vi "Initialize.vi"(8 "error in":errorcluster, 10 "InstanceName":string, 11 "Chiller Cluster - 2 Channel.lvclass":refnum<class "Cycler Cluster - 2 Channel.lvclass">) -> (0 "error out":errorcluster, 3 "output cluster":refnum<class "Cycler Cluster - 2 Channel.lvclass">)   [LabVIEW 2023, in "Cycler Cluster - 2 Channel.lvclass"]
uses:
  Cycler Cluster - 2 Channel.lvclass
  Cycler Cluster - 2 Channel.lvclass/Cycler Cluster - 2 Channel.ctl
  aa699e23-44e5-4879-a6c3-559a5ef9d2df.vi
  f052ae29-6a80-40ba-948a-362e912d77bd.vi
  293d8571-9b14-4487-9d38-5c4ef123197a.vi
  16278833-8dfa-4f0a-81f5-f65bd27da24d.vi
  da48c8f8-b897-4dcf-9451-5b341042a248.vi
  f0f9fcd1-ad99-4552-afb1-31be6853704b.vi
  aa699e23-44e5-4879-a6c3-559a5ef9d2df.vi/4bc1c15b-36ab-481f-b8dd-c64075ce723a.vi
  f052ae29-6a80-40ba-948a-362e912d77bd.vi/4bc1c15b-36ab-481f-b8dd-c64075ce723a.vi
  293d8571-9b14-4487-9d38-5c4ef123197a.vi/4bc1c15b-36ab-481f-b8dd-c64075ce723a.vi
  16278833-8dfa-4f0a-81f5-f65bd27da24d.vi/4bc1c15b-36ab-481f-b8dd-c64075ce723a.vi
  da48c8f8-b897-4dcf-9451-5b341042a248.vi/4bc1c15b-36ab-481f-b8dd-c64075ce723a.vi
  f0f9fcd1-ad99-4552-afb1-31be6853704b.vi/4bc1c15b-36ab-481f-b8dd-c64075ce723a.vi
  <vilib>/ADAS Replay HIL/AdasHilServices/AdasHilServices Fill In Error Info Ex.vi
  Utilities/Utilities.lvlib
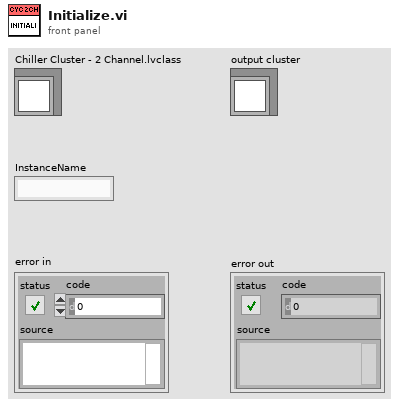
[diagram p1: front panel]
types:
  T1 = cluster{"OnOff.ACT":bool, "ErrorAcknowledge.ACT":bool, "IsoMeasurement.ACT":bool, "ParallelMode.ACT":bool}
  T2 = cluster{"OnOff.STS":i32, "Error.STS":i32, "Watchdog.STS":i32, "IsoMeasurement.STS":i32, "ParallelMode.STS":i32}
  T3 = cluster{"ErrorAcknowledge.ch01.ACT":bool, "OutputEnable.ch01.ACT":bool, "ControlMode.ch01.CTL":u16, "Voltage.ch01.SP":dbl, "VoltageMIN.ch01.SP":dbl, "VoltageMAX.ch01.SP":dbl, "VoltageGrad.ch01.SP":dbl, "Current.ch01.SP":dbl, "CurrentMIN.ch01.SP":dbl, "CurrentMAX.ch01.SP":dbl, "CurrentGrad.ch01.SP":dbl, "Power.ch01.SP":dbl, "Power.ch01.SP":dbl, "Power.ch01.SP":dbl, "PowerGrad.ch01.SP":dbl, "ParameterSet.ch01.CTL":i32}
  T4 = cluster{"Error.ch01.STS":i32, "OutputEnable.ch01.STS":i32, "ControlMode.ch01.STS":u16, "Voltage.ch01.AV":dbl, "Current.ch01.AV":dbl, "Power.ch01.AV":dbl, "VoltageNominal.ch01.AV":dbl, "CurrentNominal.ch01.AV":dbl, "PowerNominal.ch01.AV":dbl, "ParameterSet.ch01.STS":i32}
  T5 = cluster{"ErrorAcknowledge.ch02.ACT":bool, "OutputEnable.ch02.ACT":bool, "ControlMode.ch02.CTL":u16, "Voltage.ch02.SP":dbl, "VoltageMIN.ch02.SP":dbl, "VoltageMAX.ch02.SP":dbl, "VoltageGrad.ch02.SP":dbl, "Current.ch02.SP":dbl, "CurrentMIN.ch02.SP":dbl, "CurrentMAX.ch02.SP":dbl, "CurrentGrad.ch02.SP":dbl, "Power.ch02.SP":dbl, "PowerMIN.ch02.SP":dbl, "PowerMAX.ch02.SP":dbl, "PowerGrad.ch02.SP":dbl, "ParameterSet.ch02.CTL":i32}
  T6 = cluster{"Error.ch02.STS":i32, "OutputEnable.ch02.STS":i32, "ControlMode.ch02.STS":u16, "Voltage.ch02.AV":dbl, "Current.ch02.AV":dbl, "Power.ch02.AV":dbl, "VoltageNominal.ch02.AV":dbl, "CurrentNominal.ch02.AV":dbl, "PowerNominal.ch02.AV":dbl, "ParameterSet.ch02.STS":i32}
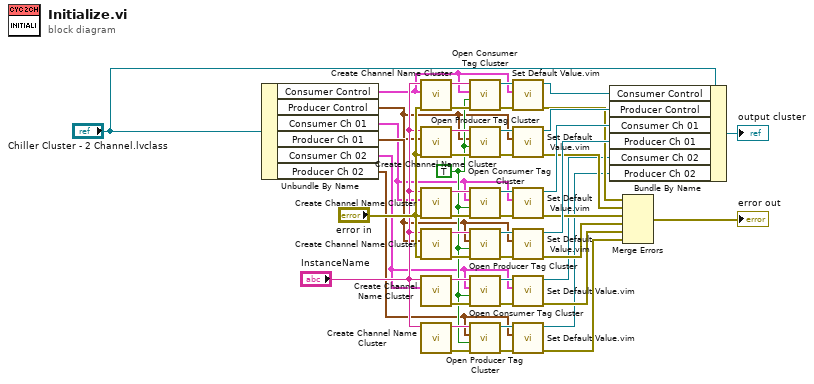
[diagram p0: block diagram]
diagram:
  w12 = TRUE ("Create if not found? (T)")
  n1 = Unbundle By Name("Chiller Cluster - 2 Channel.lvclass") -> ("Consumer Control"=w1:T1, "Producer Control"=w2:T2, "Consumer Ch 01"=w3:T3, "Producer Ch 01"=w4:T4, "Consumer Ch 02"=w5:T5, "Producer Ch 02"=w6:T6)
  n2 = call "Create Channel Name Cluster.vi"("error in"="error in", "Cluster"=w1, "Instance Name"="InstanceName") -> ("error out"=w29:errorcluster, "Data Channel Name"=w48:string)  [unwired: 7 in]
  n3 = call "Create Channel Name Cluster.vi"("error in"="error in", "Cluster"=w2, "Instance Name"="InstanceName") -> ("error out"=w30:errorcluster, "Data Channel Name"=w47:string)  [unwired: 7 in]
  n4 = call "Create Channel Name Cluster.vi"("error in"="error in", "Cluster"=w3, "Instance Name"="InstanceName") -> ("error out"=w35:errorcluster, "Data Channel Name"=w40:string)  [unwired: 7 in]
  n5 = call "Create Channel Name Cluster.vi"("error in"="error in", "Cluster"=w4, "Instance Name"="InstanceName") -> ("error out"=w33:errorcluster, "Data Channel Name"=w39:string)  [unwired: 7 in]
  n6 = call "Create Channel Name Cluster.vi"("Cluster"=w5, "Instance Name"="InstanceName") -> ("error out"=w18:errorcluster, "Data Channel Name"=w14:string)  [unwired: 8 in]
  n7 = call "Create Channel Name Cluster.vi"("Instance Name"="InstanceName") -> ("error out"=w16:errorcluster, "Data Channel Name"=w21:string)  [unwired: 9 in]
  n8 = call "Open Consumer Tag Cluster.vi"("error in"=w29, "Create if not found? (T)"=w12, "Cluster"=w1, "Channel Name"=w48) -> ("error out"=w44:errorcluster, "ADAS HIL Channel"=w46:refnum<k21>)  [unwired: 6 in]
  n9 = call "Open Producer Tag Cluster.vi"("error in"=w30, "Create if not found? (T)"=w12, "Cluster"=w2, "Channel Name"=w47) -> ("error out"=w43:errorcluster, "ADAS HIL Channel"=w42:refnum<k21>)  [unwired: 6 in]
  n10 = call "Open Consumer Tag Cluster.vi"("error in"=w35, "Create if not found? (T)"=w12, "Cluster"=w3, "Channel Name"=w40) -> ("error out"=w36:errorcluster, "ADAS HIL Channel"=w37:refnum<k21>)  [unwired: 6 in]
  n11 = call "Open Producer Tag Cluster.vi"("error in"=w33, "Create if not found? (T)"=w12, "Cluster"=w4, "Channel Name"=w39) -> ("error out"=w34:errorcluster, "ADAS HIL Channel"=w38:refnum<k21>)  [unwired: 6 in]
  n12 = call "Open Consumer Tag Cluster.vi"("error in"=w18, "Create if not found? (T)"=w12, "Cluster"=w5, "Channel Name"=w14) -> ("error out"=w19:errorcluster, "ADAS HIL Channel"=w13:refnum<k21>)  [unwired: 6 in]
  n13 = call "Open Producer Tag Cluster.vi"("error in"=w16, "Create if not found? (T)"=w12, "Cluster"=w6, "Channel Name"=w21) -> ("error out"=w17:errorcluster, "ADAS HIL Channel"=w20:refnum<k21>)  [unwired: 6 in]
  n14 = call "Set Default Value.vim"("error in"=w44, "Data in"=w1, "ADAS HIL Channel in"=w46) -> ("error out"=w27:errorcluster, "ADAS HIL Channel out"=w45:refnum<k21>)  [unwired: 7 in]
  n15 = call "Set Default Value.vim"("error in"=w43, "Data in"=w2, "ADAS HIL Channel in"=w42) -> ("error out"=w26:errorcluster, "ADAS HIL Channel out"=w41:refnum<k21>)  [unwired: 7 in]
  n16 = call "Set Default Value.vim"("error in"=w36, "Data in"=w3, "ADAS HIL Channel in"=w37) -> ("error out"=w25:errorcluster, "ADAS HIL Channel out"=w32:refnum<k21>)  [unwired: 7 in]
  n17 = call "Set Default Value.vim"("error in"=w34, "Data in"=w4, "ADAS HIL Channel in"=w38) -> ("error out"=w24:errorcluster, "ADAS HIL Channel out"=w31:refnum<k21>)  [unwired: 7 in]
  n18 = call "Set Default Value.vim"("error in"=w19, "Data in"=w5, "ADAS HIL Channel in"=w13) -> ("error out"=w11:errorcluster, "ADAS HIL Channel out"=w9:refnum<k21>)  [unwired: 7 in]
  n19 = call "Set Default Value.vim"("error in"=w17, "Data in"=w6, "ADAS HIL Channel in"=w20) -> ("error out"=w10:errorcluster, "ADAS HIL Channel out"=w8:refnum<k21>)  [unwired: 7 in]
  n20 = Bundle By Name(cluster="Chiller Cluster - 2 Channel.lvclass", "Consumer Control"=w45, "Producer Control"=w41, "Consumer Ch 01"=w32, "Producer Ch 01"=w31, "Consumer Ch 02"=w9, "Producer Ch 02"=w8) -> (→"output cluster":refnum<class "Cycler Cluster - 2 Channel.lvclass">)
  n21 = Merge Errors(w27, w26, w25, w24, w11, w10) -> (→"error out":errorcluster)
